vi "PositionSaveFGV.vi"(6 "Image Cluster Input":T1, 7 "PositionSave Commands":T3=enum."NewList", 8 "Error In":errorcluster, 9 "CompleteTableString":string[][](array[string]), 10 "Table Index":i32, 11 "Position Data In":T4) -> (0 "Error Out":errorcluster, 1 "SavedImage out":T2, 2 "cancelled/failed":bool, 3 "Position Data Out":string[][](array[string]), 4 "Path":path)   [LabVIEW 2012]
doc: "SciScan 1.2 160622\nThis FGV implements the core functionality of the 'position save module'.\n\nFunctinality implemented:\n* Create a new position data file\n* Loading an existing position file\n* Updating the position file by adding (appending) a new"
uses:
  Custom Control and Typedefs/PositionData.ctl
  PositionSaveFGVCommands.ctl
  <vilib>/vision/Image Controls.llb/IMAQ Image.ctl
  Custom Control and Typedefs/ImageCluster.ctl
  Folder and Path Creation_Commands.ctl
  CommonResource VIs/File IO/File_In_Use__Commands.ctl
  ImageIO_commands.ctl
  <vilib>/Utility/file.llb/Write To Spreadsheet File (string).vi
  <vilib>/Utility/file.llb/Read From Spreadsheet File (string).vi
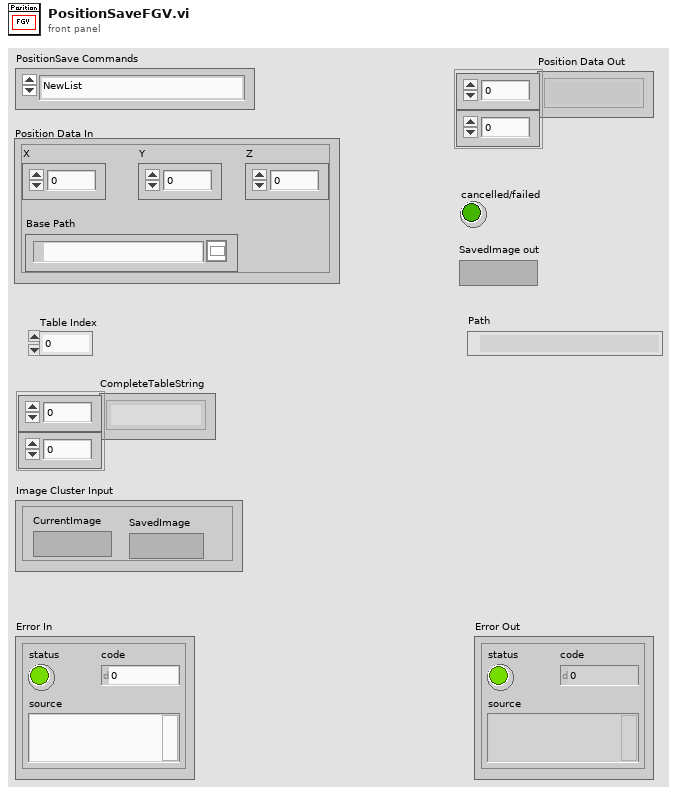
[diagram p1: front panel]
types:
  T1 = typedef "ImageCluster.ctl" = cluster{"CurrentImage":T2, "SavedImage":T2}
  T2 = typedef "IMAQ Image.ctl" = refnum<image>
  T3 = typedef "PositionSaveFGVCommands.ctl" = enum16{"Initialize", "NewList", "LoadList", "CopyList", "DeleteSelected", "SetPosition", "SetNewOrigin", "UpdateEntireTable", "GetPosition", "Shutdown and Cleanup"}
  T4 = typedef "PositionData.ctl" = cluster{"X":dbl, "Y":dbl, "Z":dbl, "Base Path":path}
  T5 = typedef "Folder and Path Creation_Commands.ctl" = enum16{"New Position File", "Load Position File", "Copy Position File"}
  T6 = typedef "File_In_Use__Commands.ctl" = enum16{"IsFileInUse?", "IsFolderInUse?"}
  T7 = enum16{"open", "replace", "create", "open or create", "replace or create", "replace or create with confirmation"}
  T8 = typedef "ImageIO_commands.ctl" = enum16{"ReadImage", "WriteImage"}
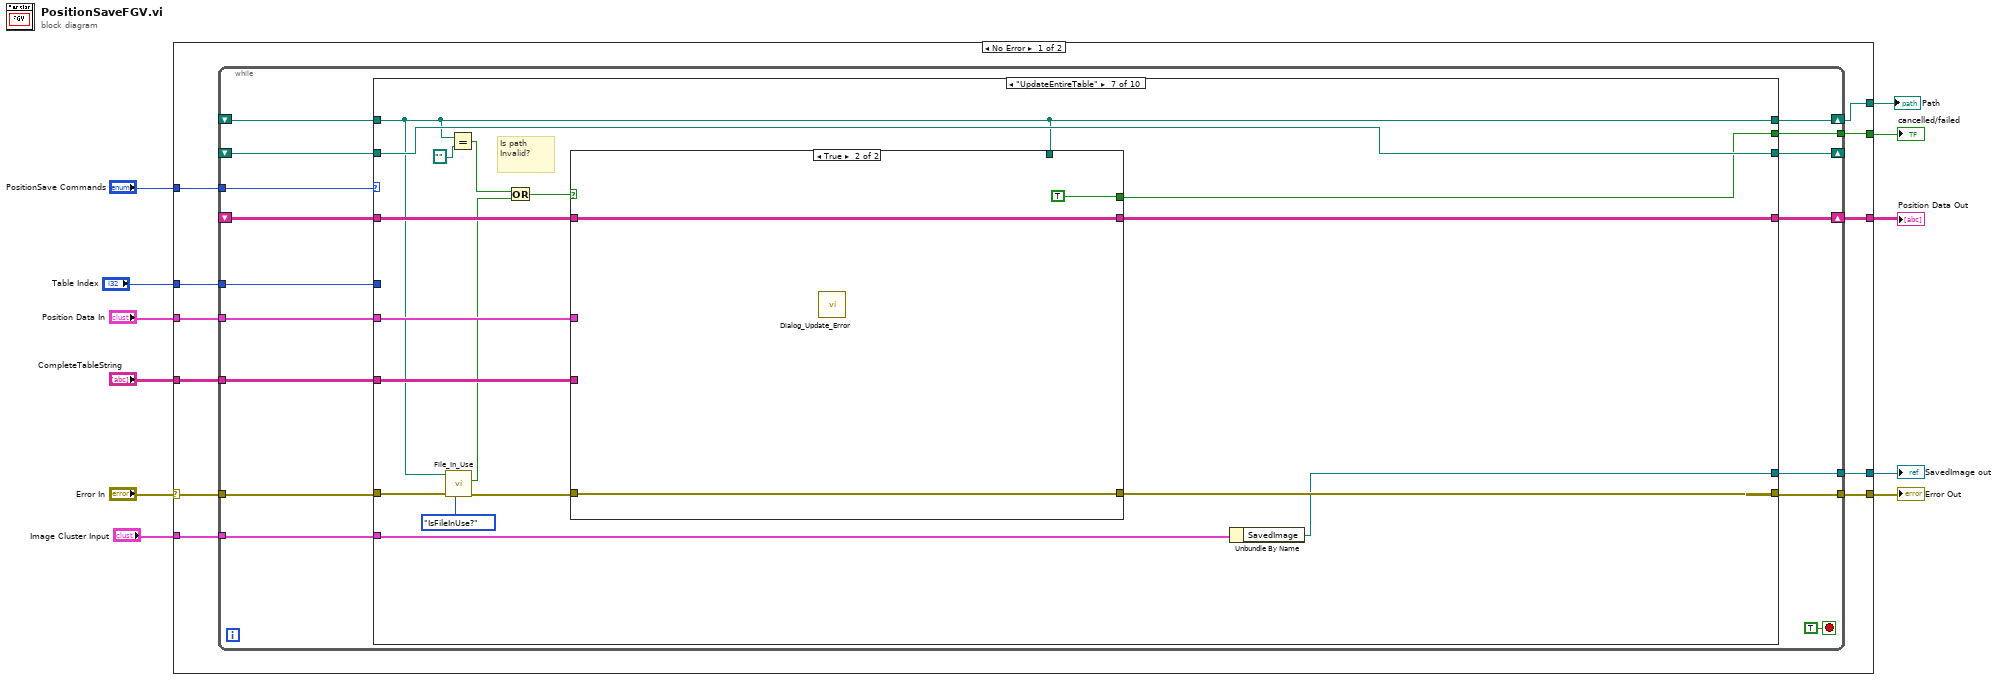
[diagram p0: block diagram]
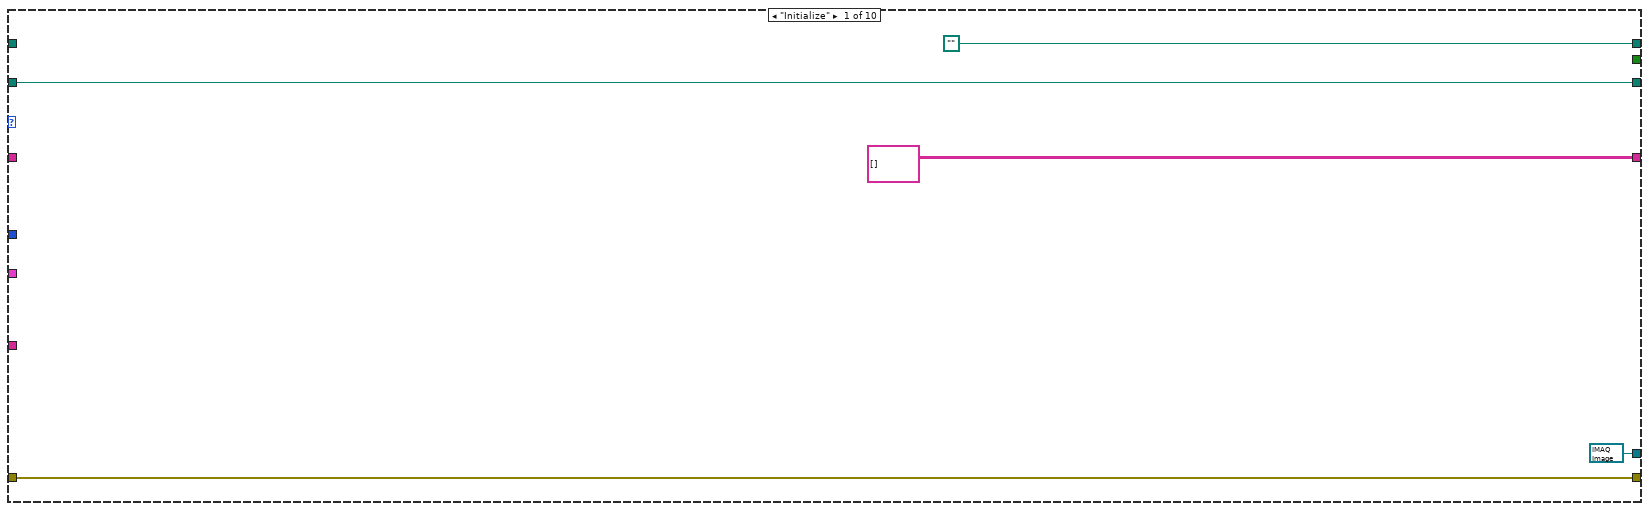
[diagram p2: hidden frame]
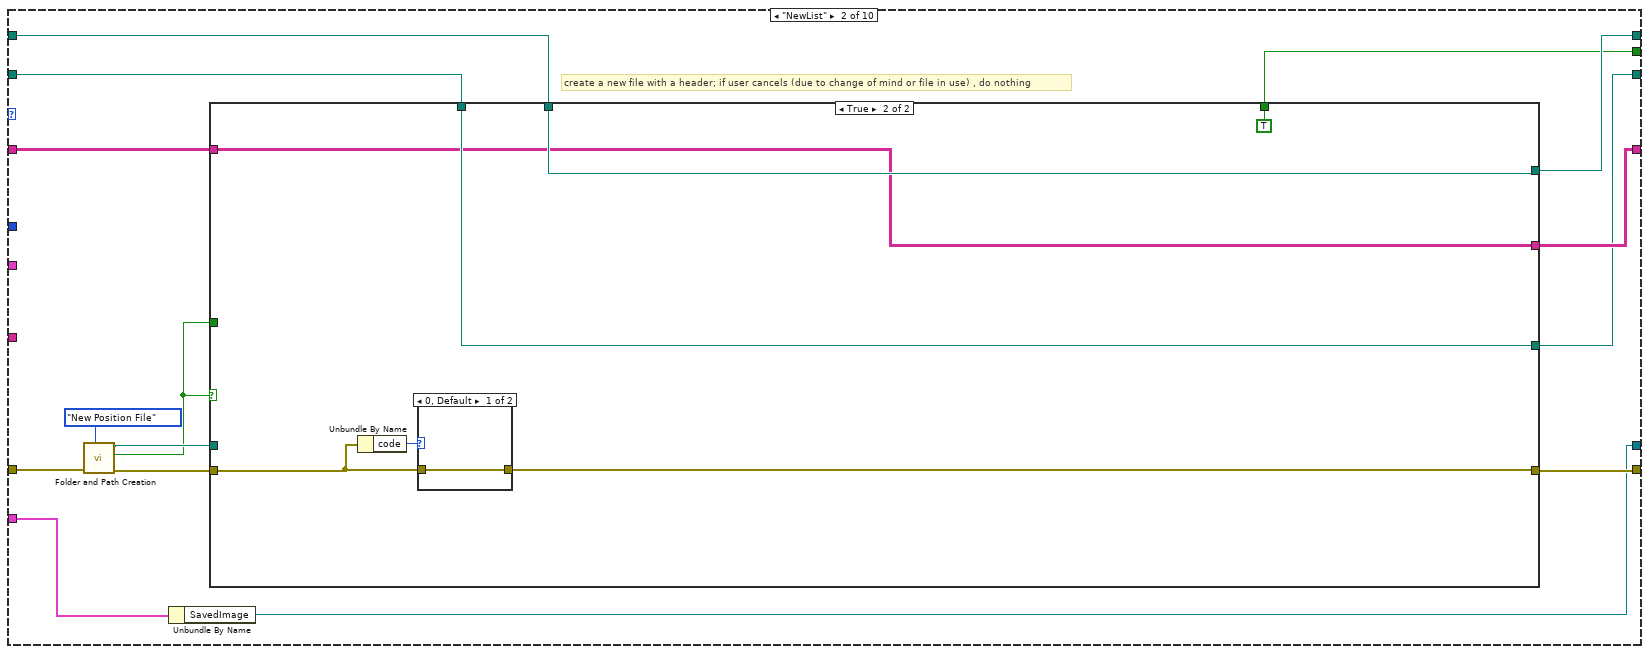
[diagram p3: hidden frame]
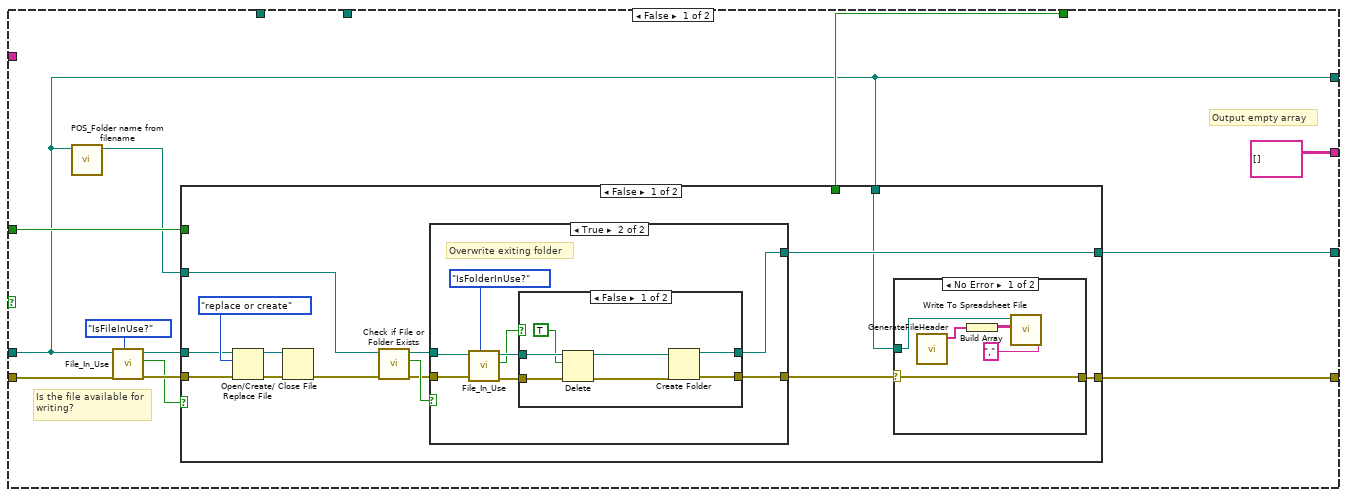
[diagram p4: hidden frame]
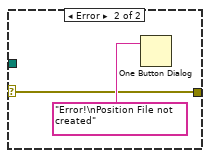
[diagram p5: hidden frame]
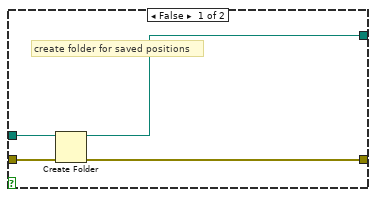
[diagram p6: hidden frame]
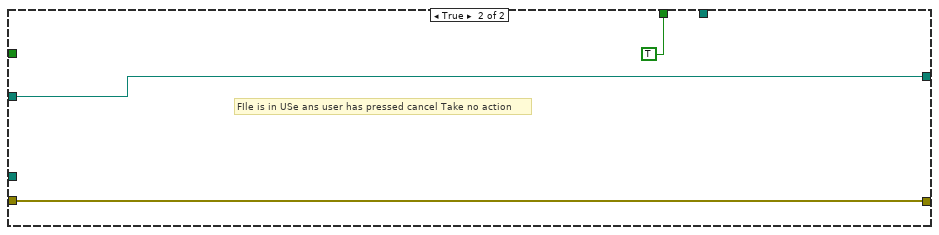
[diagram p8: hidden frame]
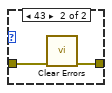
[diagram p9: hidden frame]
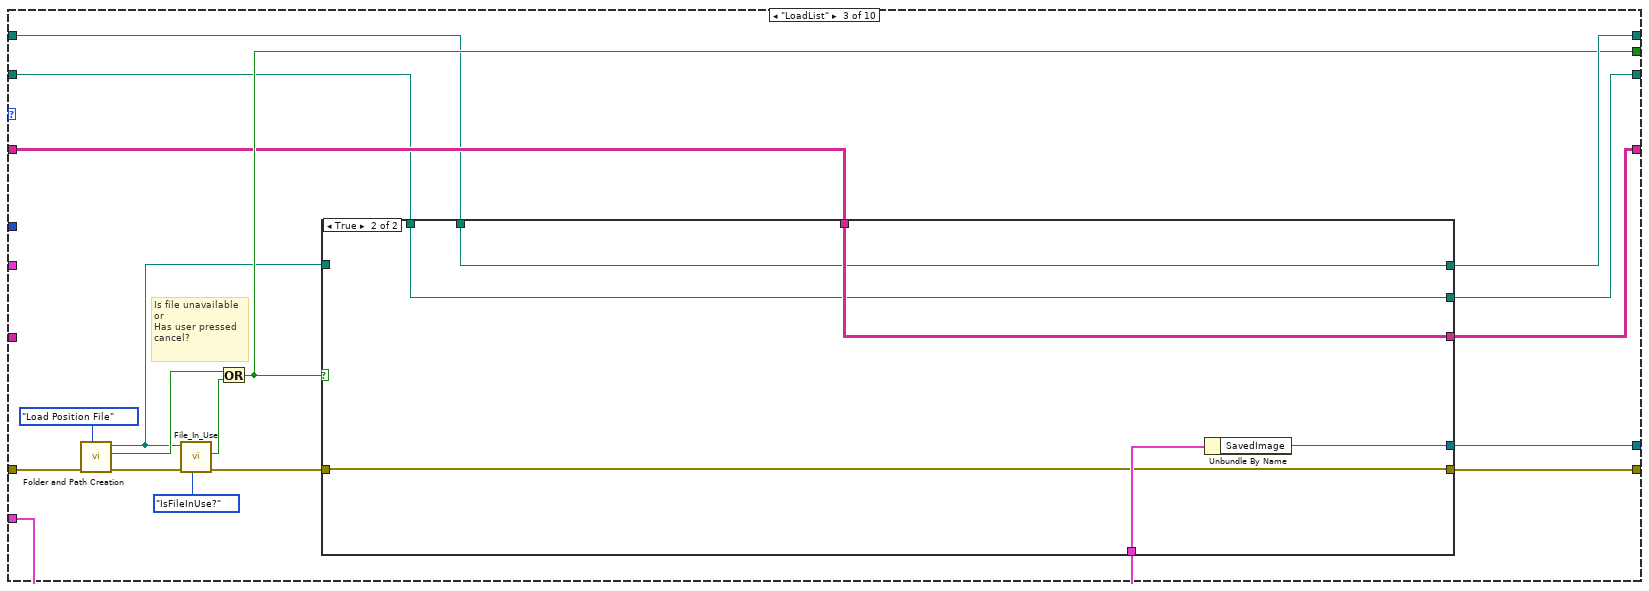
[diagram p10: hidden frame]
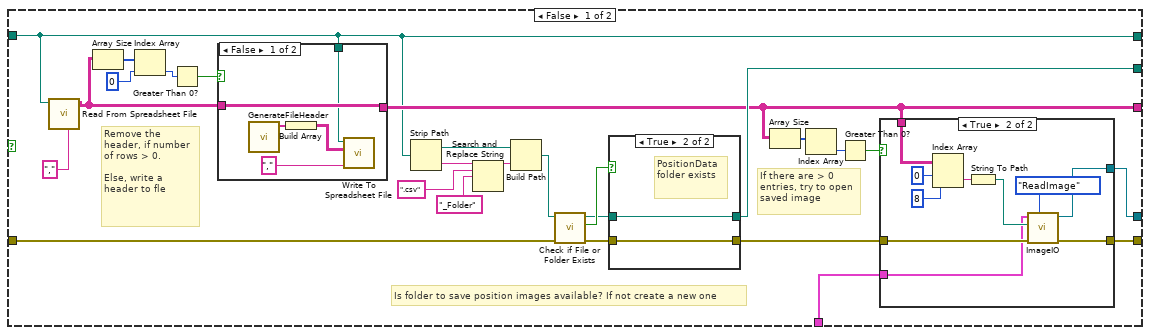
[diagram p11: hidden frame]
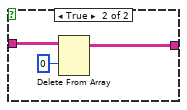
[diagram p12: hidden frame]
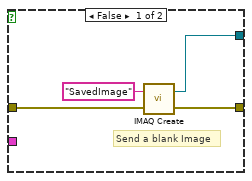
[diagram p13: hidden frame]
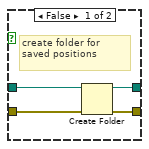
[diagram p14: hidden frame]
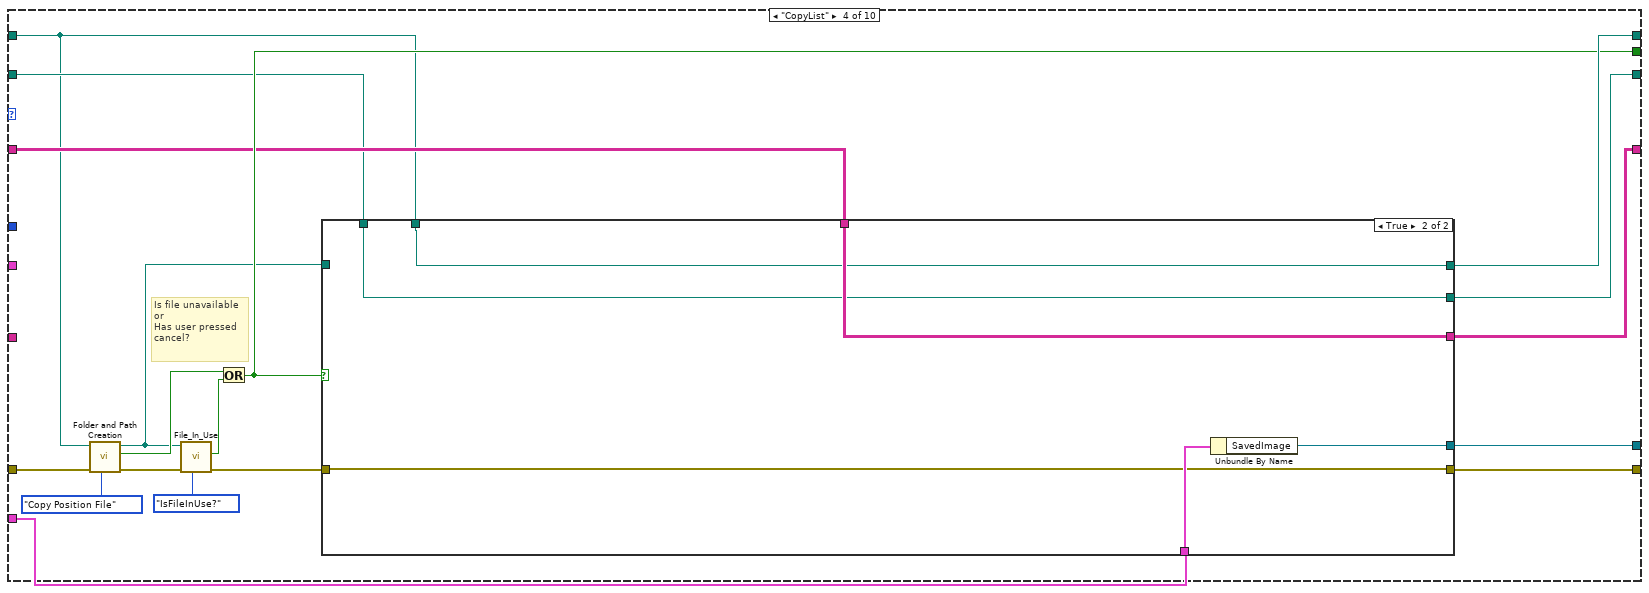
[diagram p15: hidden frame]
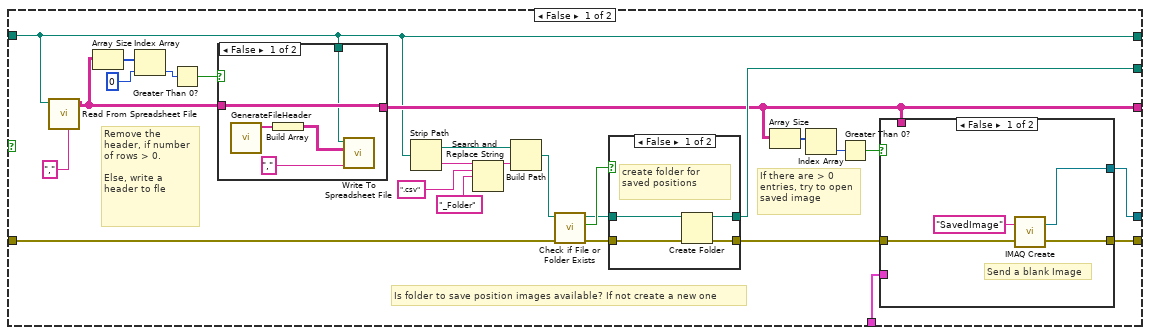
[diagram p16: hidden frame]
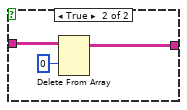
[diagram p17: hidden frame]
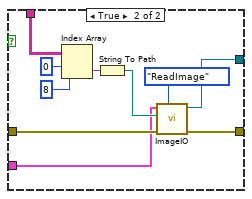
[diagram p18: hidden frame]
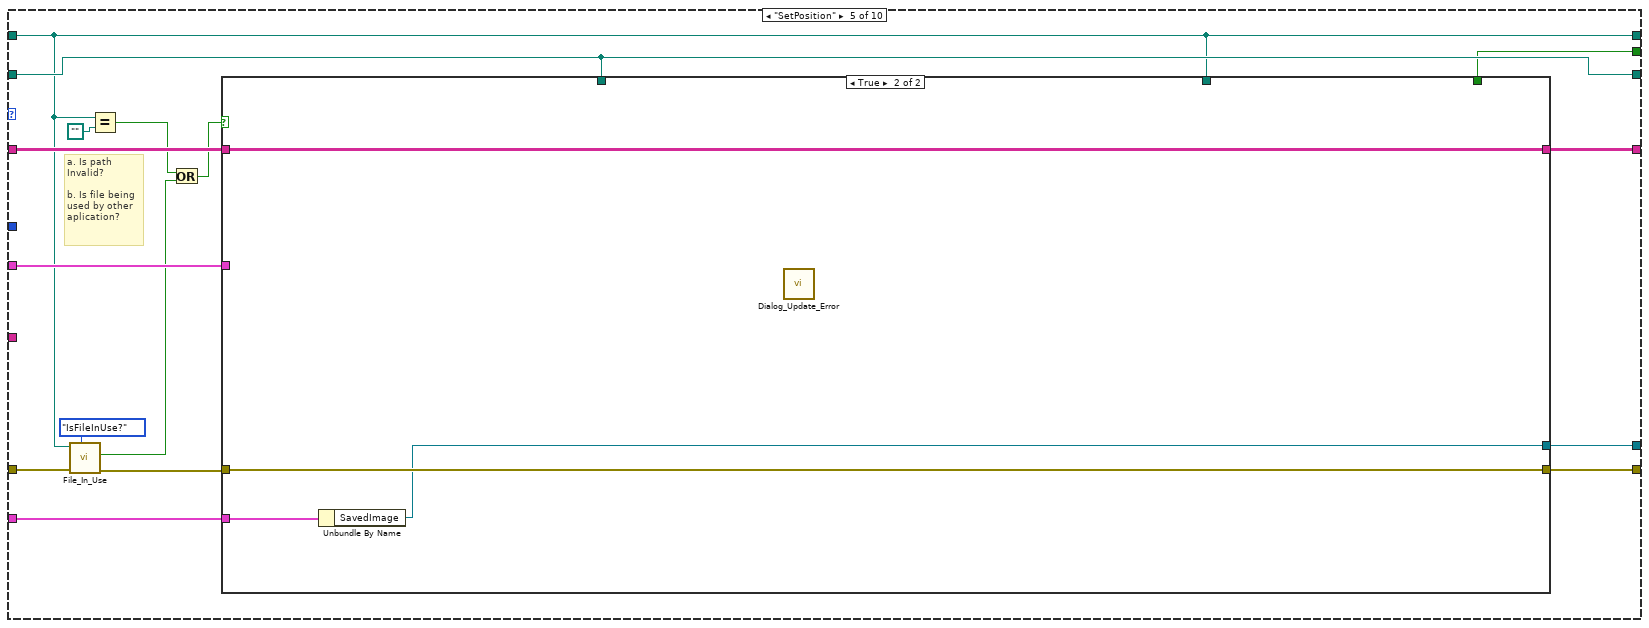
[diagram p20: hidden frame]
diagram:
  n1 = case shown="No Error" "Error In" {
    selector: "Error In" -> [w20 w606]
    tunnel: "PositionSave Commands" -> [w22 _]
    tunnel: "Position Data In" -> [w21 _]
    tunnel: [w19 w606] -> w8
    tunnel: [w18 string[][] [] ("all rows")] -> w7
    tunnel: [w17 _] -> w6
    tunnel: "CompleteTableString" -> [w16 _]
    tunnel: "Table Index" -> [w15 _]
    tunnel: [w14 w602] -> w3
    tunnel: "Image Cluster Input" -> [w13 w603]
    tunnel: [w12 path ""] -> w1
    frame No Error {
      n2 = while {
        tunnel: w22 -> [w37]
        shift-right: [w36] -> w18
        shift-left: _ -> [w35]
        tunnel: w21 -> [w34]
        shift-right: [w33] -> w12
        shift-left: _ -> [w32]
        tunnel: w20 -> [w31]
        tunnel: [w30] -> w19
        tunnel: [w29] -> w17
        tunnel: w16 -> [w28]
        tunnel: w15 -> [w27]
        shift-right: [w26] -> _
        shift-left: _ -> [w25]
        tunnel: [w24] -> w14
        tunnel: w13 -> [w23]
        stop <- TRUE stop-if-true
        n3 = case shown="\"UpdateEntireTable\"" w37 {
          tunnel: [string[][] [] ("all rows") w57 w143 w221 w295 w389 w503 w533 w549 string[][] [] ("all rows")] -> w36
          tunnel: w35 -> [_ w44 w128 w206 w296 w390 w504 w533 w551 _]
          tunnel: w34 -> [_ _ _ _ w297 w391 w505 _ _ _]
          tunnel: [path "" w56 w141 w219 w285 w379 w494 w534 w548 path ""] -> w33
          tunnel: w32 -> [_ w47 w127 w204 w285 w379 w494 w534 w544 _]
          tunnel: [w41 w58 w142 w220 w293 w387 w501 w532 w537 w601] -> w30
          tunnel: w31 -> [w41 w55 w140 w218 w287 w382 w493 w532 w545 w601]
          tunnel: [_ w52 w133 w211 w289 w383 w489 _ w538 _] -> w29
          tunnel: w28 -> [_ _ _ _ _ _ w500 _ _ _]
          tunnel: w27 -> [_ _ _ _ _ _ _ _ w550 _]
          tunnel: [w40 w54 w139 w217 w291 w386 w499 w531 w547 w598] -> w26
          tunnel: w25 -> [w40 w46 w126 w205 w291 w386 w499 w531 w547 w598]
          tunnel: [T2 refnum ("SavedImage") w45 w137 w215 w292 w385 w497 w529 w535 T2 refnum ("SavedImage")] -> w24
          tunnel: w23 -> [_ w53 w138 w216 w290 w384 w498 w530 w536 _]
          frame "Initialize" {
          }
          frame "NewList" {
            # "create a new file with a header; if user cancels (due to change of mind or file in use) , do nothing"
            n4 = call "Folder and Path Creation.vi"("Action"=Folder_and_Path_Creation_Commands."New Position File", "Error In"=w55) -> ("Error Out"=w51:errorcluster, "Cancelled?"=w48:bool, "CSV File path"=w49:path)  [unwired: 7 in]
            n5 = Unbundle By Name(w53) -> ("SavedImage"=w45:T2)
            n6 = case shown="True" w48 {
              tunnel: w51 -> [w66 w121]
              tunnel: w49 -> [w60 _]
              tunnel: [w68 w120] -> w58
              tunnel: [w60 w118] -> w56
              tunnel: [string[][] [] w116] -> w57
              tunnel: [w69 w117] -> w54
              tunnel: w48 -> [w64 _]
              tunnel: [w63 TRUE] -> w52
              tunnel: w47 -> [_ w118]
              tunnel: w46 -> [_ w117]
              tunnel: w44 -> [_ w116]
              frame False {
                # "Is the file available for\nwriting?"
                # "Output empty array"
                n7 = call "POS_Folder name from filename.vi"("File Path In"=w60) -> ("Folder Path Out"=w59:path)  [unwired: 10 in]
                n8 = call "File_In_Use.vi"("Action"=File_In_Use__Commands."IsFileInUse?", "Error In"=w66, "Path IN"=w60) -> ("Error Out"=w65:errorcluster, "Cancelled?"=w61:bool, "Path OUT"=w62:path)  [unwired: 5 in, 1 out]
                n9 = case shown="False" w61 {
                  tunnel: w59 -> [w75 w115]
                  tunnel: [w81 w115] -> w69
                  tunnel: [w80 w114] -> w68
                  tunnel: w60 -> [w78 _]
                  tunnel: w65 -> [w76 w114]
                  tunnel: w64 -> [_ _]
                  tunnel: [_ TRUE] -> w63
                  tunnel: w62 -> [w71 _]
                  frame False {
                    n10 = Open/Create/Replace File(file path (use dialog)=w71, error in=w76, operation (0:open)=T7."replace or create") -> (refnum out=w73:refnum<file>, error out=w74:errorcluster)  [unwired: 3 in, 1 out]
                    n11 = Close File(refnum=w73, error in=w74) -> (error out=w72:errorcluster)  [unwired: 1 out]
                    n12 = call <vilib>:"Check if File or Folder Exists.vi"("error in (no error)"=w72, "path"=w75) -> ("error out"=w82:errorcluster, "file or folder exists?"=w84:bool, "dup path"=w83:path)  [unwired: 7 in]
                    n13 = case shown="True" w84 {
                      tunnel: w83 -> [w93 w101]
                      tunnel: w82 -> [w95 w102]
                      tunnel: [w94 w96] -> w79
                      tunnel: [w92 w103] -> w81
                      frame False {
                        # "create folder for saved positions"
                        n14 = Create Folder(path (use dialog)=w93, error in=w95) -> (created path=w92:path, error out=w94:errorcluster)  [unwired: 1 in, 1 out]
                      }
                      frame True {
                        # "Overwrite exiting folder"
                        n15 = call "File_In_Use.vi"("Action"=File_In_Use__Commands."IsFolderInUse?", "Error In"=w102, "Path IN"=w101) -> ("Error Out"=w98:errorcluster, "Cancelled?"=w97:bool, "Path OUT"=w100:path)  [unwired: 5 in, 1 out]
                        n16 = case shown="False" w97 {
                          tunnel: w98 -> [w106 w111]
                          tunnel: [w110 w111] -> w96
                          tunnel: [w109 w112] -> w103
                          tunnel: w100 -> [w108 w112]
                          frame False {
                            n17 = Delete(path (use dialog)=w108, entire hierarchy (F)=TRUE, error in=w106) -> (deleted path=w104:path, error out=w105:errorcluster)  [unwired: 2 in, 1 out]
                            n18 = Create Folder(path (use dialog)=w104, error in=w105) -> (created path=w109:path, error out=w110:errorcluster)  [unwired: 1 in, 1 out]
                          }
                          frame True {
                          }
                        }
                      }
                    }
                    n19 = case shown="No Error" w79 {
                      selector: w79 -> [w86 w90]
                      tunnel: w78 -> [w88 _]
                      tunnel: [w86 w90] -> w80
                      frame No Error {
                        n20 = call "GenerateFileHeader.vi"() -> ("Position File Header"=w85:string[])  [unwired: 11 in]
                        n21 = Build Array(w85) -> (w89:string[][])
                        n22 = call-poly <vilib>:"Write To Spreadsheet File.vi"("delimiter (\\t)"="," ("delimiter (\\t)"), "2D data"=w89, "file path (dialog if empty)"=w88) -> ()  [unwired: 5 in, 1 out]
                      }
                      frame Error {
                        n23 = One Button Dialog(message="Error!\nPosition File not created") -> ()  [unwired: 1 in, 1 out]
                      }
                    }
                  }
                  frame True {
                    # "FIle is in USe ans user has pressed cancel Take no action"
                  }
                }
              }
              frame True {
                n24 = Unbundle By Name(w121) -> ("code"=w122:i32)
                n25 = case shown="0, Default" w122 {
                  tunnel: w121 -> [w123 w125]
                  tunnel: [w123 w124] -> w120
                  frame 0, Default {
                  }
                  frame 43 {
                    n26 = call <vilib>:"Clear Errors.vi"("error in (no error)"=w125) -> ("error out"=w124:errorcluster)  [unwired: 6 in]
                  }
                }
              }
            }
          }
          frame "LoadList" {
            # "Is file unavailable\nor \nHas user pressed\ncancel?"
            n27 = call "Folder and Path Creation.vi"("Action"=Folder_and_Path_Creation_Commands."Load Position File", "Error In"=w140) -> ("Error Out"=w131:errorcluster, "Cancelled?"=w130:bool, "CSV File path"=w129:path)  [unwired: 7 in]
            n28 = call "File_In_Use.vi"("Action"=File_In_Use__Commands."IsFileInUse?", "Error In"=w131, "Path IN"=w129) -> ("Error Out"=w136:errorcluster, "Cancelled?"=w135:bool)  [unwired: 5 in, 2 out]
            n29 = Or(x=w130, y=w135) -> (x .or. y?=w133:bool)
            n30 = case shown="True" w133 {
              tunnel: w129 -> [w145 _]
              tunnel: [w158 w201] -> w143
              tunnel: w136 -> [w166 w200]
              tunnel: [w160 w200] -> w142
              tunnel: [w145 w199] -> w141
              tunnel: [w162 w198] -> w139
              tunnel: w138 -> [w157 w203]
              tunnel: [w159 w202] -> w137
              tunnel: w128 -> [_ w201]
              tunnel: w127 -> [_ w199]
              tunnel: w126 -> [_ w198]
              frame False {
                # "If there are > 0\nentries, try to open\nsaved image"
                # "Is folder to save position images available? If not create a new one"
                # "Remove the header, if number of rows > 0.\n\nElse, write a header to fle"
                n31 = call-poly <vilib>:"Read From Spreadsheet File.vi"("delimiter (\\t)"="," ("delimiter (\\t)"), "file path (dialog if empty)"=w145) -> ("all rows"=w144:string[][])  [unwired: 5 in, 4 out]
                n32 = Array Size(array=w144) -> (size(s)=w156:i32[])
                n33 = Index Array(array=w156, index=0) -> (element=w154:i32)
                n34 = Greater Than 0?(x=w154) -> (x > 0?=w153:bool)
                n35 = case shown="False" w153 {
                  tunnel: w144 -> [w174 w177]
                  tunnel: [w174 w175] -> w158
                  tunnel: w145 -> [w173 _]
                  frame False {
                    n36 = call "GenerateFileHeader.vi"() -> ("Position File Header"=w170:string[])  [unwired: 11 in]
                    n37 = Build Array(w170) -> (w172:string[][])
                    n38 = call-poly <vilib>:"Write To Spreadsheet File.vi"("delimiter (\\t)"="," ("delimiter (\\t)"), "2D data"=w172, "file path (dialog if empty)"=w173) -> ()  [unwired: 5 in, 1 out]
                  }
                  frame True {
                    n39 = Delete From Array(array=w177, index (row)=0) -> (array with subset deleted=w175:string[][])  [unwired: 2 in, 1 out]
                  }
                }
                n40 = Strip Path(path=w145) -> (stripped path=w152:path, name=w151:string)
                n41 = Search and Replace String(input string=w151, search string=".csv", replace string="_Folder" ("replace string (\"\")")) -> (result string=w148:string)  [unwired: 5 in, 3 out]
                n42 = Build Path(base path=w152, name or relative path=w148) -> (appended path=w147:path)
                n43 = call <vilib>:"Check if File or Folder Exists.vi"("error in (no error)"=w166, "path"=w147) -> ("error out"=w167:errorcluster, "file or folder exists?"=w169:bool, "dup path"=w168:path)  [unwired: 7 in]
                n44 = case shown="True" w169 {
                  tunnel: w168 -> [w193 w196]
                  tunnel: w167 -> [w195 w197]
                  tunnel: [w194 w197] -> w161
                  tunnel: [w192 w196] -> w162
                  frame False {
                    # "create folder for saved positions"
                    n45 = Create Folder(path (use dialog)=w193, error in=w195) -> (created path=w192:path, error out=w194:errorcluster)  [unwired: 1 in, 1 out]
                  }
                  frame True {
                    # "PositionData folder exists"
                  }
                }
                n46 = Array Size(array=w158) -> (size(s)=w165:i32[])
                n47 = Index Array(array=w165) -> (element=w164:i32)  [unwired: 1 in]
                n48 = Greater Than 0?(x=w164) -> (x > 0?=w163:bool)
                n49 = case shown="True" w163 {
                  tunnel: w161 -> [w181 w187]
                  tunnel: [w180 w182] -> w160
                  tunnel: [w179 w184] -> w159
                  tunnel: w158 -> [_ w191]
                  tunnel: w157 -> [_ w185]
                  frame False {
                    # "Send a blank Image"
                    n50 = call "IMAQ Create"("Image Name"="SavedImage", "error in (no error)"=w181) -> ("New Image"=w179:T2, "error out"=w180:errorcluster)  [unwired: 3 in]
                  }
                  frame True {
                    n51 = Index Array(array=w191, index (row)=0, index (col)=8 ("disabled index (col)")) -> (element=w188:string)
                    n52 = String To Path(string=w188) -> (path=w186:path)
                    n53 = call "ImageIO.vi"("Pos_ImageIO_commands"=ImageIO_commands."ReadImage", "Error In"=w187, "Image File Path"=w186, "ImageCluster IN"=w185) -> ("Error Out"=w182:errorcluster, "Saved Image OUT"=w184:T2)  [unwired: 5 in, 1 out]
                  }
                }
              }
              frame True {
                n54 = Unbundle By Name(w203) -> ("SavedImage"=w202:T2)
              }
            }
          }
          frame "CopyList" {
            # "Is file unavailable\nor \nHas user pressed\ncancel?"
            n55 = call "Folder and Path Creation.vi"("Action"=Folder_and_Path_Creation_Commands."Copy Position File", "Error In"=w218, "Source Path for Copy"=w204) -> ("Error Out"=w209:errorcluster, "Cancelled?"=w208:bool, "CSV File path"=w207:path)  [unwired: 6 in]
            n56 = call "File_In_Use.vi"("Action"=File_In_Use__Commands."IsFileInUse?", "Error In"=w209, "Path IN"=w207) -> ("Error Out"=w214:errorcluster, "Cancelled?"=w213:bool)  [unwired: 5 in, 2 out]
            n57 = Or(x=w208, y=w213) -> (x .or. y?=w211:bool)
            n58 = case shown="True" w211 {
              tunnel: w207 -> [w223 _]
              tunnel: [w236 w279] -> w221
              tunnel: w214 -> [w244 w278]
              tunnel: [w238 w278] -> w220
              tunnel: [w223 w277] -> w219
              tunnel: [w240 w276] -> w217
              tunnel: w216 -> [w235 w281]
              tunnel: [w237 w280] -> w215
              tunnel: w206 -> [_ w279]
              tunnel: w205 -> [_ w276]
              tunnel: w204 -> [_ w277]
              frame False {
                # "If there are > 0\nentries, try to open\nsaved image"
                # "Is folder to save position images available? If not create a new one"
                # "Remove the header, if number of rows > 0.\n\nElse, write a header to fle"
                n59 = call-poly <vilib>:"Read From Spreadsheet File.vi"("delimiter (\\t)"="," ("delimiter (\\t)"), "file path (dialog if empty)"=w223) -> ("all rows"=w222:string[][])  [unwired: 5 in, 4 out]
                n60 = Array Size(array=w222) -> (size(s)=w234:i32[])
                n61 = Index Array(array=w234, index=0) -> (element=w232:i32)
                n62 = Greater Than 0?(x=w232) -> (x > 0?=w231:bool)
                n63 = case shown="False" w231 {
                  tunnel: w222 -> [w252 w255]
                  tunnel: [w252 w253] -> w236
                  tunnel: w223 -> [w251 _]
                  frame False {
                    n64 = call "GenerateFileHeader.vi"() -> ("Position File Header"=w248:string[])  [unwired: 11 in]
                    n65 = Build Array(w248) -> (w250:string[][])
                    n66 = call-poly <vilib>:"Write To Spreadsheet File.vi"("delimiter (\\t)"="," ("delimiter (\\t)"), "2D data"=w250, "file path (dialog if empty)"=w251) -> ()  [unwired: 5 in, 1 out]
                  }
                  frame True {
                    n67 = Delete From Array(array=w255, index (row)=0) -> (array with subset deleted=w253:string[][])  [unwired: 2 in, 1 out]
                  }
                }
                n68 = Strip Path(path=w223) -> (stripped path=w230:path, name=w229:string)
                n69 = Search and Replace String(input string=w229, search string=".csv", replace string="_Folder" ("replace string (\"\")")) -> (result string=w226:string)  [unwired: 5 in, 3 out]
                n70 = Build Path(base path=w230, name or relative path=w226) -> (appended path=w225:path)
                n71 = call <vilib>:"Check if File or Folder Exists.vi"("error in (no error)"=w244, "path"=w225) -> ("error out"=w245:errorcluster, "file or folder exists?"=w247:bool, "dup path"=w246:path)  [unwired: 7 in]
                n72 = case shown="False" w247 {
                  tunnel: w246 -> [w271 w274]
                  tunnel: w245 -> [w273 w275]
                  tunnel: [w272 w275] -> w239
                  tunnel: [w270 w274] -> w240
                  frame False {
                    # "create folder for saved positions"
                    n73 = Create Folder(path (use dialog)=w271, error in=w273) -> (created path=w270:path, error out=w272:errorcluster)  [unwired: 1 in, 1 out]
                  }
                  frame True {
                    # "PositionData folder exists"
                  }
                }
                n74 = Array Size(array=w236) -> (size(s)=w243:i32[])
                n75 = Index Array(array=w243) -> (element=w242:i32)  [unwired: 1 in]
                n76 = Greater Than 0?(x=w242) -> (x > 0?=w241:bool)
                n77 = case shown="False" w241 {
                  tunnel: w239 -> [w259 w265]
                  tunnel: [w258 w260] -> w238
                  tunnel: [w257 w262] -> w237
                  tunnel: w236 -> [_ w269]
                  tunnel: w235 -> [_ w263]
                  frame False {
                    # "Send a blank Image"
                    n78 = call "IMAQ Create"("Image Name"="SavedImage", "error in (no error)"=w259) -> ("New Image"=w257:T2, "error out"=w258:errorcluster)  [unwired: 3 in]
                  }
                  frame True {
                    n79 = Index Array(array=w269, index (row)=0, index (col)=8 ("disabled index (col)")) -> (element=w266:string)
                    n80 = String To Path(string=w266) -> (path=w264:path)
                    n81 = call "ImageIO.vi"("Pos_ImageIO_commands"=ImageIO_commands."ReadImage", "Error In"=w265, "Image File Path"=w264, "ImageCluster IN"=w263) -> ("Error Out"=w260:errorcluster, "Saved Image OUT"=w262:T2)  [unwired: 5 in, 1 out]
                  }
                }
              }
              frame True {
                n82 = Unbundle By Name(w281) -> ("SavedImage"=w280:T2)
              }
            }
          }
          frame "SetPosition" {
            # "a. Is path Invalid?\n\nb. Is file being used by other aplication?"
            n83 = call "File_In_Use.vi"("Action"=File_In_Use__Commands."IsFileInUse?", "Error In"=w287, "Path IN"=w285) -> ("Error Out"=w286:errorcluster, "Cancelled?"=w282:bool)  [unwired: 5 in, 2 out]
            n84 = Equal?(x=w285, y=path "") -> (x = y?=w284:bool)
            n85 = Or(x=w284, y=w282) -> (x .or. y?=w283:bool)
            n86 = case shown="True" w283 {
              tunnel: w285 -> [w307 _]
              tunnel: w297 -> [w333 _]
              tunnel: w296 -> [w309 w375]
              tunnel: [w306 w375] -> w295
              tunnel: w286 -> [w312 w374]
              tunnel: [w305 w374] -> w293
              tunnel: w290 -> [w315 w373]
              tunnel: [w304 w372] -> w292
              tunnel: w291 -> [w316 _]
              tunnel: [w302 _] -> w289
              frame False {
                w337 = i16 4 ("precision (6)")
                w345 = 0.0 ("number")
                w349 = i16 4 ("precision (6)")
                # "Current X, Y, Z"
                # "X, Y, Z of origin"
                # "Build file path"
                # "2. Calulate the Relative X, Y and Z"
                # "XRel"
                # "YRel"
                # "ZRel"
                # "Timestamp"
                # "Notes"
                # "Image Path"
                # "1. Generate a Row for insertion into the spreadsheet"
                # "3. Insert new position at the end and write to spreadsheet file; if image save succeeds"
                n87 = Unbundle By Name(w333) -> ("X"=w359:dbl, "Y"=w358:dbl, "Z"=w357:dbl)
                n88 = Get Date/Time In Seconds() -> (seconds since 1Jan1904=w319:timestamp)
                n89 = Path To String(path=path "") -> (string=w348:string)
                n90 = Format Date/Time String(seconds (now)=w319) -> (date/time string=w350:string)  [unwired: 2 in]
                n91 = Number To Fractional String(number=w359, precision (6)=w349) -> (F-format string=w356:string)  [unwired: 2 in]
                n92 = Number To Fractional String(number=w358, precision (6)=w349) -> (F-format string=w355:string)  [unwired: 2 in]
                n93 = Number To Fractional String(number=w357, precision (6)=w349) -> (F-format string=w354:string)  [unwired: 2 in]
                n94 = Number To Fractional String(number=w345, precision (6)=w349) -> (F-format string=w353:string)  [unwired: 2 in]
                n95 = Number To Fractional String(number=w345, precision (6)=w349) -> (F-format string=w352:string)  [unwired: 2 in]
                n96 = Number To Fractional String(number=w345, precision (6)=w349) -> (F-format string=w351:string)  [unwired: 2 in]
                n97 = Build Array(w356, w355, w354, w353, w352, w351, w350, "" ("element"), w348) -> (w332:string[])
                n98 = Index Array(array=w309, index (row)=0) -> (element=w334:string[])  [unwired: 1 in]
                n99 = Index Array(array=w334) -> (element #1=w342:string, element #2=w343:string, element #3=w344:string)  [unwired: 3 in]
                n100 = Format Date/Time String(time format string (%c)="POS_%Y%m%d__%H_%M_%S%3u", seconds (now)=w319) -> (date/time string=w299:string)  [unwired: 1 in]
                n101 = Fract/Exp String To Number(string=w342) -> (number=w329:dbl)  [unwired: 3 in, 1 out]
                n102 = Fract/Exp String To Number(string=w343) -> (number=w326:dbl)  [unwired: 3 in, 1 out]
                n103 = Fract/Exp String To Number(string=w344) -> (number=w323:dbl)  [unwired: 3 in, 1 out]
                n104 = Unbundle By Name(w333) -> ("X"=w330:dbl, "Y"=w327:dbl, "Z"=w324:dbl)
                n105 = Search and Replace String(input string=w299, search string=".", replace string="_" ("replace string (\"\")")) -> (result string=w298:string)  [unwired: 5 in, 3 out]
                n106 = Subtract(x=w330, y=w329) -> (x-y=w328:dbl)
                n107 = Subtract(x=w327, y=w326) -> (x-y=w325:dbl)
                n108 = Subtract(x=w324, y=w323) -> (x-y=w322:dbl)
                n109 = Concatenate Strings(w298, ".PNG" ("string")) -> (w321:string)
                n110 = Number To Fractional String(number=w328, precision (6)=w337) -> (F-format string=w340:string)  [unwired: 2 in]
                n111 = Number To Fractional String(number=w325, precision (6)=w337) -> (F-format string=w338:string)  [unwired: 2 in]
                n112 = Number To Fractional String(number=w322, precision (6)=w337) -> (F-format string=w331:string)  [unwired: 2 in]
                n113 = Build Path(base path=w316, name or relative path=w321) -> (appended path=w313:path)
                n114 = Path To String(path=w313) -> (string=w314:string)
                n115 = Replace Array Subset(array=w332, new element #1=w340, index #1=3 ("index"), new element #2=w338, index #2=4 ("index"), new element #3=w331, index #3=5 ("index"), new element #4=w314, index #4=8 ("index")) -> (w308:string[])
                n116 = call "ImageIO.vi"("Pos_ImageIO_commands"=ImageIO_commands."WriteImage", "Error In"=w312, "Image File Path"=w313, "ImageCluster IN"=w315) -> ("Error Out"=w311:errorcluster, "Error!"=w310:bool, "Saved Image OUT"=w304:T2)  [unwired: 5 in]
                n117 = case shown="False" w310 {
                  tunnel: w311 -> [w365 w369]
                  tunnel: w309 -> [w366 w371]
                  tunnel: w308 -> [w363 _]
                  tunnel: w307 -> [w364 _]
                  tunnel: [w362 w371] -> w306
                  tunnel: [w365 w369] -> w305
                  tunnel: [_ TRUE] -> w302
                  frame False {
                    # "New 2 D array to\nwrite to file"
                    # "Append to 2D array"
                    n118 = Insert Into Array(array=w366, new element=w363) -> (w362:string[][])  [unwired: 2 in]
                    n119 = call "GenerateFileHeader.vi"() -> ("Position File Header"=w360:string[])  [unwired: 11 in]
                    n120 = Build Array (concatenate)(w360, w362) -> (w361:string[][])
                    n121 = call-poly <vilib>:"Write To Spreadsheet File.vi"("delimiter (\\t)"="," ("delimiter (\\t)"), "2D data"=w361, "file path (dialog if empty)"=w364) -> ()  [unwired: 5 in, 1 out]
                  }
                  frame True {
                    n122 = One Button Dialog(message="Set position failed!") -> ()  [unwired: 1 in, 1 out]
                  }
                }
              }
              frame True {
                n123 = Unbundle By Name(w373) -> ("SavedImage"=w372:T2)
                n124 = call "Dialog_Update_Error.vi"() -> ()  [unwired: 12 in]
              }
            }
          }
          frame "SetNewOrigin" {
            # "Is path Invalid?"
            n125 = call "File_In_Use.vi"("Action"=File_In_Use__Commands."IsFileInUse?", "Error In"=w382, "Path IN"=w379) -> ("Error Out"=w381:errorcluster, "Cancelled?"=w378:bool)  [unwired: 5 in, 2 out]
            n126 = Equal?(x=w379, y=path "") -> (x = y?=w377:bool)
            n127 = Or(x=w377, y=w378) -> (x .or. y?=w376:bool)
            n128 = case shown="True" w376 {
              tunnel: w379 -> [w426 _]
              tunnel: w391 -> [w409 _]
              tunnel: w390 -> [w408 w488]
              tunnel: [w400 w488] -> w389
              tunnel: w381 -> [w397 w487]
              tunnel: [w394 w487] -> w387
              tunnel: w386 -> [w405 _]
              tunnel: [w395 w484] -> w385
              tunnel: w384 -> [w398 w485]
              tunnel: [w392 TRUE] -> w383
              frame False {
                w410 = 0.0 ("number")
                w414 = i16 4 ("precision (6)")
                # "2. If  save image succeeds, try to write the .csv file. If either of the two fails, set the cancelled/failed indicator to TRUE"
                # "1. Generate the image path and try to save image in the designated folder"
                # "Try to save the image"
                # "Error while saving images?"
                # "Build image file path"
                # "Timestamp"
                # "XRel"
                # "YRel"
                # "ZRel"
                # "Image Path"
                # "Notes"
                n129 = Get Date/Time In Seconds() -> (seconds since 1Jan1904=w407:timestamp)
                n130 = Format Date/Time String(time format string (%c)="POS_%Y%m%d__%H_%M_%S", seconds (now)=w407) -> (date/time string=w403:string)  [unwired: 1 in]
                n131 = Unbundle By Name(w409) -> ("X"=w425:dbl, "Y"=w424:dbl, "Z"=w423:dbl)
                n132 = Concatenate Strings(w403, ".PNG" ("string")) -> (w404:string)
                n133 = Format Date/Time String(seconds (now)=w407) -> (date/time string=w416:string)  [unwired: 2 in]
                n134 = Build Path(base path=w405, name or relative path=w404) -> (appended path=w399:path)
                n135 = Path To String(path=path "") -> (string=w413:string)
                n136 = Number To Fractional String(number=w425, precision (6)=w414) -> (F-format string=w422:string)  [unwired: 2 in]
                n137 = Number To Fractional String(number=w424, precision (6)=w414) -> (F-format string=w421:string)  [unwired: 2 in]
                n138 = Number To Fractional String(number=w423, precision (6)=w414) -> (F-format string=w420:string)  [unwired: 2 in]
                n139 = Number To Fractional String(number=w410, precision (6)=w414) -> (F-format string=w419:string)  [unwired: 2 in]
                n140 = Number To Fractional String(number=w410, precision (6)=w414) -> (F-format string=w418:string)  [unwired: 2 in]
                n141 = Number To Fractional String(number=w410, precision (6)=w414) -> (F-format string=w417:string)  [unwired: 2 in]
                n142 = call "ImageIO.vi"("Pos_ImageIO_commands"=ImageIO_commands."WriteImage", "Error In"=w397, "Image File Path"=w399, "ImageCluster IN"=w398) -> ("Error Out"=w394:errorcluster, "Error!"=w396:bool, "Saved Image OUT"=w395:T2)  [unwired: 5 in]
                n143 = Build Array(w422, w421, w420, w419, w418, w417, w416, "" ("element"), w413) -> (w415:string[])
                n144 = Path To String(path=w399) -> (string=w401:string)
                n145 = case shown="False" w396 {
                  tunnel: w426 -> [w448 _]
                  tunnel: w415 -> [w444 _]
                  tunnel: w409 -> [w443 _]
                  tunnel: w408 -> [w442 w483]
                  tunnel: w401 -> [w439 _]
                  tunnel: [w434 w483] -> w400
                  tunnel: [FALSE TRUE] -> w392
                  frame False {
                    w438 = 0 ("index (row)")
                    # "If an empty array,\ninsert into array;\nelse, replace"
                    # "Insert a default note"
                    # "Add header & write to file"
                    n146 = for {
                      tunnel: w442 -> [w471] mode=indexing
                      tunnel: w443 -> [w481]
                      tunnel: [w464] -> w431 mode=indexing
                      w466 = i16 4 ("precision (6)")
                      # "Calulate the ABSOLUTE X, Y and Z for every entry"
                      n147 = Index Array(array=w471, index #1=3 ("index"), index #2=4 ("index"), index #3=5 ("index")) -> (element #1=w478:string, element #2=w479:string, element #3=w480:string)
                      n148 = Unbundle By Name(w481) -> ("X"=w476:dbl, "Y"=w474:dbl, "Z"=w473:dbl)
                      n149 = Fract/Exp String To Number(string=w478) -> (number=w477:dbl)  [unwired: 3 in, 1 out]
                      n150 = Fract/Exp String To Number(string=w479) -> (number=w475:dbl)  [unwired: 3 in, 1 out]
                      n151 = Fract/Exp String To Number(string=w480) -> (number=w472:dbl)  [unwired: 3 in, 1 out]
                      n152 = Add(x=w477, y=w476) -> (x+y=w459:dbl)
                      n153 = Add(x=w475, y=w474) -> (x+y=w458:dbl)
                      n154 = Add(x=w472, y=w473) -> (x+y=w457:dbl)
                      n155 = Number To Fractional String(number=w459, precision (6)=w466) -> (F-format string=w469:string)  [unwired: 2 in]
                      n156 = Number To Fractional String(number=w458, precision (6)=w466) -> (F-format string=w467:string)  [unwired: 2 in]
                      n157 = Number To Fractional String(number=w457, precision (6)=w466) -> (F-format string=w463:string)  [unwired: 2 in]
                      n158 = Replace Array Subset(array=w471, new element #1=w469, index #1=0 ("index"), new element #2=w467, index #2=1 ("index"), new element #3=w463, index #3=2 ("index")) -> (w464:string[])
                    }
                    n159 = Array Size(array=w431) -> (size(s)=w430:i32[])
                    n160 = Index Array(array=w430, index=0) -> (element=w428:i32)
                    n161 = Greater Than 0?(x=w428) -> (x > 0?=w427:bool)
                    n162 = case shown="True" w427 {
                      tunnel: w444 -> [w452 w456]
                      tunnel: w431 -> [w450 w454]
                      tunnel: [w449 w453] -> w436
                      frame True {
                        # "Replace \nat row# 0"
                        n163 = Replace Array Subset(array=w450, new element=w452, index (row)=0) -> (w449:string[][])  [unwired: 1 in]
                      }
                      frame False {
                        # "Insert \nat row# 0"
                        n164 = Insert Into Array(array=w454, index (row)=0, new element=w456) -> (w453:string[][])  [unwired: 1 in]
                      }
                    }
                    n165 = Replace Array Subset(array=w436, new element="This is the  origin" ("String"), index (row)=w438, index (col)=7 ("disabled index (col)")) -> (w435:string[][])
                    n166 = call "GenerateFileHeader.vi"() -> ("Position File Header"=w432:string[])  [unwired: 11 in]
                    n167 = Replace Array Subset(array=w435, new element=w439, index (row)=w438, index (col)=8) -> (w434:string[][])
                    n168 = Build Array (concatenate)(w432, w434) -> (w445:string[][])
                    n169 = call-poly <vilib>:"Write To Spreadsheet File.vi"("delimiter (\\t)"="," ("delimiter (\\t)"), "append to file? (new file:F)"=FALSE, "2D data"=w445, "file path (dialog if empty)"=w448) -> ()  [unwired: 4 in, 1 out]
                  }
                  frame True {
                    # "Error has occured!\nDonot write the csv file or update the 2D data array"
                    n170 = call "Dialog_Update_Error.vi"() -> ()  [unwired: 12 in]
                  }
                }
              }
              frame True {
                n171 = Unbundle By Name(w485) -> ("SavedImage"=w484:T2)
                n172 = call "Dialog_Update_Error.vi"() -> ()  [unwired: 12 in]
              }
            }
          }
          frame "UpdateEntireTable" {
            # "Is path Invalid?"
            n173 = call "File_In_Use.vi"("Action"=File_In_Use__Commands."IsFileInUse?", "Error In"=w493, "Path IN"=w494) -> ("Error Out"=w492:errorcluster, "Cancelled?"=w495:bool)  [unwired: 5 in, 2 out]
            n174 = Equal?(x=w494, y=path "") -> (x = y?=w491:bool)
            n175 = Or(x=w491, y=w495) -> (x .or. y?=w490:bool)
            n176 = case shown="True" w490 {
              tunnel: w494 -> [w520 _]
              tunnel: w505 -> [_ _]
              tunnel: w504 -> [_ w528]
              tunnel: [w513 w528] -> w503
              tunnel: w492 -> [w517 w527]
              tunnel: [w517 w527] -> w501
              tunnel: w500 -> [w510 _]
              tunnel: [_ TRUE] -> w489
              frame False {
                # "Replace any commas\nfrom Notes - this would\nmess up the CSV table"
                # "Include header"
                # "Overwrite spreadsheet file"
                n177 = Index Array(array=w510, index (col)=7 ("disabled index (col)")) -> (element=w511:string[])  [unwired: 1 in]
                n178 = for {
                  tunnel: w511 -> [w522] mode=indexing
                  tunnel: [w521] -> w508 mode=indexing
                  n179 = Search and Replace String(replace all?=TRUE ("replace all? (F)"), input string=w522, search string=",", replace string=";" ("replace string (\"\")")) -> (result string=w521:string)  [unwired: 4 in, 3 out]
                }
                n180 = call "GenerateFileHeader.vi"() -> ("Position File Header"=w506:string[])  [unwired: 11 in]
                n181 = Replace Array Subset(array=w510, new element=w508, index (col)=7 ("disabled index (col)")) -> (w507:string[][])  [unwired: 1 in]
                n182 = Build Array (concatenate)(w506, w507) -> (w516:string[][])
                n183 = call-poly <vilib>:"Write To Spreadsheet File.vi"("delimiter (\\t)"="," ("delimiter (\\t)"), "append to file? (new file:F)"=FALSE, "2D data"=w516, "file path (dialog if empty)"=w520) -> ()  [unwired: 4 in, 1 out]
                n184 = Delete From Array(array=w516, length=1, index (row)=0) -> (array with subset deleted=w513:string[][])  [unwired: 1 in, 1 out]
              }
              frame True {
                n185 = call "Dialog_Update_Error.vi"() -> ()  [unwired: 12 in]
              }
            }
            n186 = Unbundle By Name(w498) -> ("SavedImage"=w497:T2)
          }
          frame "GetPosition", Default {
            n187 = Unbundle By Name(w530) -> ("SavedImage"=w529:T2)
          }
          frame "DeleteSelected" {
            n188 = call "File_In_Use.vi"("Action"=File_In_Use__Commands."IsFileInUse?", "Error In"=w545, "Path IN"=w544) -> ("Error Out"=w541:errorcluster, "File/Folder not found"=w542:bool, "Cancelled?"=w543:bool, "Path OUT"=w539:path)  [unwired: 5 in]
            n189 = Or(x=w543, y=w542) -> (x .or. y?=w540:bool)
            n190 = case shown="True" w540 {
              tunnel: w551 -> [w563 w594]
              tunnel: w550 -> [w562 _]
              tunnel: [w553 w594] -> w549
              tunnel: [w575 w595] -> w548
              tunnel: w541 -> [w570 w596]
              tunnel: w539 -> [w574 w595]
              tunnel: [w556 w596] -> w537
              tunnel: [FALSE TRUE] -> w538
              tunnel: w536 -> [w557 w592]
              tunnel: [w555 w591] -> w535
              frame False {
                # "Add a header to the data before writing\nto file"
                # "Read path of previous image"
                # "Delete image file if found and file not in use"
                # "Update file"
                n191 = Index Array(array=w563, index (row)=w562, index (col)=8 ("disabled index (col)")) -> (element=w572:string)
                n192 = String To Path(string=w572) -> (path=w571:path)
                n193 = call <vilib>:"Check if File or Folder Exists.vi"("error in (no error)"=w570, "path"=w571) -> ("error out"=w567:errorcluster, "file or folder exists?"=w569:bool, "dup path"=w568:path)  [unwired: 7 in]
                n194 = case shown="True" w569 {
                  tunnel: w568 -> [_ w581]
                  tunnel: w567 -> [w579 w584]
                  tunnel: [w579 w586] -> w564
                  frame False {
                  }
                  frame True {
                    n195 = call "File_In_Use.vi"("Action"=File_In_Use__Commands."IsFileInUse?", "Error In"=w584, "Path IN"=w581) -> ("Error Out"=w583:errorcluster, "Cancelled?"=w582:bool, "Path OUT"=w580:path)  [unwired: 5 in, 1 out]
                    n196 = case shown="False" w582 {
                      tunnel: [w589 w590] -> w586
                      tunnel: w583 -> [w588 w590]
                      tunnel: w580 -> [w587 _]
                      frame False {
                        n197 = Delete(path (use dialog)=w587, error in=w588) -> (error out=w589:errorcluster)  [unwired: 3 in, 2 out]
                      }
                      frame True {
                      }
                    }
                  }
                }
                n198 = Delete From Array(array=w563, length=1, index (row)=w562) -> (array with subset deleted=w553:string[][])  [unwired: 1 in, 1 out]
                n199 = Decrement(x=w562) -> (x-1=w561:i32)
                n200 = Index Array(array=w563, index (row)=w561, index (col)=8 ("disabled index (col)")) -> (element=w560:string)
                n201 = String To Path(string=w560) -> (path=w558:path)
                n202 = call "GenerateFileHeader.vi"() -> ("Position File Header"=w554:string[])  [unwired: 11 in]
                n203 = Build Array (concatenate)(w554, w553) -> (w552:string[][])
                n204 = call "ImageIO.vi"("Pos_ImageIO_commands"=ImageIO_commands."ReadImage", "Error In"=w564, "Image File Path"=w558, "ImageCluster IN"=w557) -> ("Error Out"=w556:errorcluster, "Saved Image OUT"=w555:T2)  [unwired: 5 in, 1 out]
                n205 = call-poly <vilib>:"Write To Spreadsheet File.vi"("delimiter (\\t)"="," ("delimiter (\\t)"), "append to file? (new file:F)"=FALSE, "2D data"=w552, "file path (dialog if empty)"=w574) -> ("new file path (Not A Path if cancelled)"=w575:path)  [unwired: 4 in]
              }
              frame True {
                n206 = Unbundle By Name(w592) -> ("SavedImage"=w591:T2)
                n207 = call "Dialog_Update_Error.vi"() -> ()  [unwired: 12 in]
              }
            }
          }
          frame "Shutdown and Cleanup" {
          }
        }
      }
    }
    frame Error {
      n208 = Unbundle By Name(w603) -> ("SavedImage"=w602:T2)
    }
  }
  "Error Out" <- w8
  "Position Data Out" <- w7
  "cancelled/failed" <- w6
  "SavedImage out" <- w3
  "Path" <- w1
